vi "EvaluateCave.vi"(9 "Small Cave Visited Twize In":bool, 10 "Path(Caves)":refnum<class "12_Cave.lvclass">[](array[class]), 11 "Cave":refnum<class "12_Cave.lvclass">) -> (1 "Small Cave Visited Twize Out":bool, 2 "Stop":bool, 3 "End Found":bool)   [LabVIEW 2020, in "2021_12.lvclass"]
uses:
  2021_12.lvclass
  45103e70-66f0-4670-8e98-666914fd66a7.vi
  12_Cave_class/12_Cave.lvclass
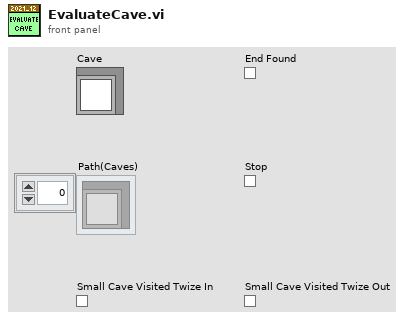
[diagram p1: front panel]
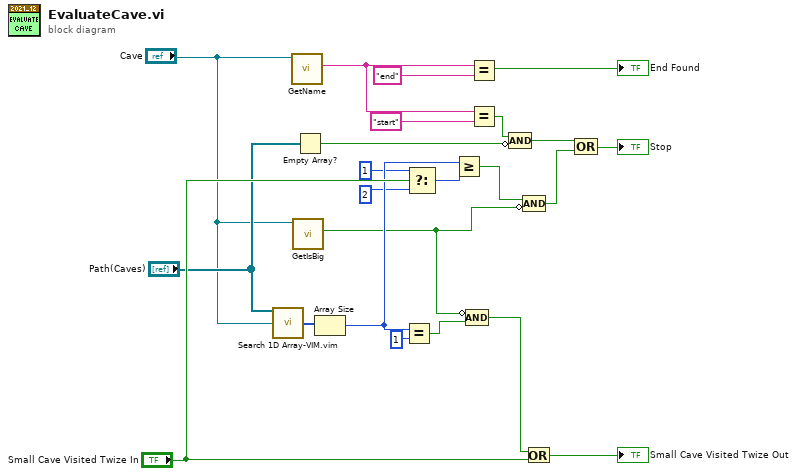
[diagram p0: block diagram]
diagram:
  n1 = call "Search 1D Array-VIM.vim"("Array"="Path(Caves)", "Element Data"="Cave") -> ("Indices of Elements"=w4:i32[])  [unwired: 7 in]
  n2 = call-dynamic "GetName.vi"("reference in"="Cave") -> ("Name"=w6:string)  [unwired: 8 in, 2 out]
  n3 = call-dynamic "GetIsBig.vi"("reference in"="Cave") -> ("Is Big"=w16:bool)  [unwired: 8 in, 2 out]
  n4 = Empty Array?(array="Path(Caves)") -> (empty?=w7:bool)
  n5 = Array Size(array=w4) -> (size(s)=w18:i32)
  n6 = Equal?(x=w18, y=1 ("t")) -> (x = y?=w20:bool)
  n7 = Select(t=1, s="Small Cave Visited Twize In", f=2 ("t")) -> (s? t:f=w12:i32)
  n8 = Greater Or Equal?(x=w18, y=w12) -> (x >= y?=w11:bool)
  n9 = Compound Arithmetic op=AND(invert w16, w20) -> (w21:bool)
  n10 = Equal?(x=w6, y="end") -> (x = y?=→"End Found":bool)
  n11 = Equal?(x=w6, y="start") -> (x = y?=w8:bool)
  n12 = Compound Arithmetic op=AND(w8, invert w7) -> (w9:bool)
  n13 = Compound Arithmetic op=AND(w11, invert w16) -> (w10:bool)
  n14 = Or(x=w21, y="Small Cave Visited Twize In") -> (x .or. y?=→"Small Cave Visited Twize Out":bool)
  n15 = Compound Arithmetic op=OR(w9, w10) -> (→"Stop":bool)
